vi "serial_communication.vi"() -> ()   [LabVIEW 2017]
uses:
  Utility Sub VIs/diode_charts.ctl
  <vilib>/Instr/_visa.llb/VISA Set IO Buffer Mask.ctl
  <vilib>/Instr/_visa.llb/VISA Flush IO Buffer Mask.ctl
  <vilib>/Instr/_visa.llb/VISA Configure Serial Port (Instr).vi
panel:
  out "read buffer":string
  in  "stop":bool
  in  "VISA resource name":refnum<visa-resource-name>
  out "value":T1
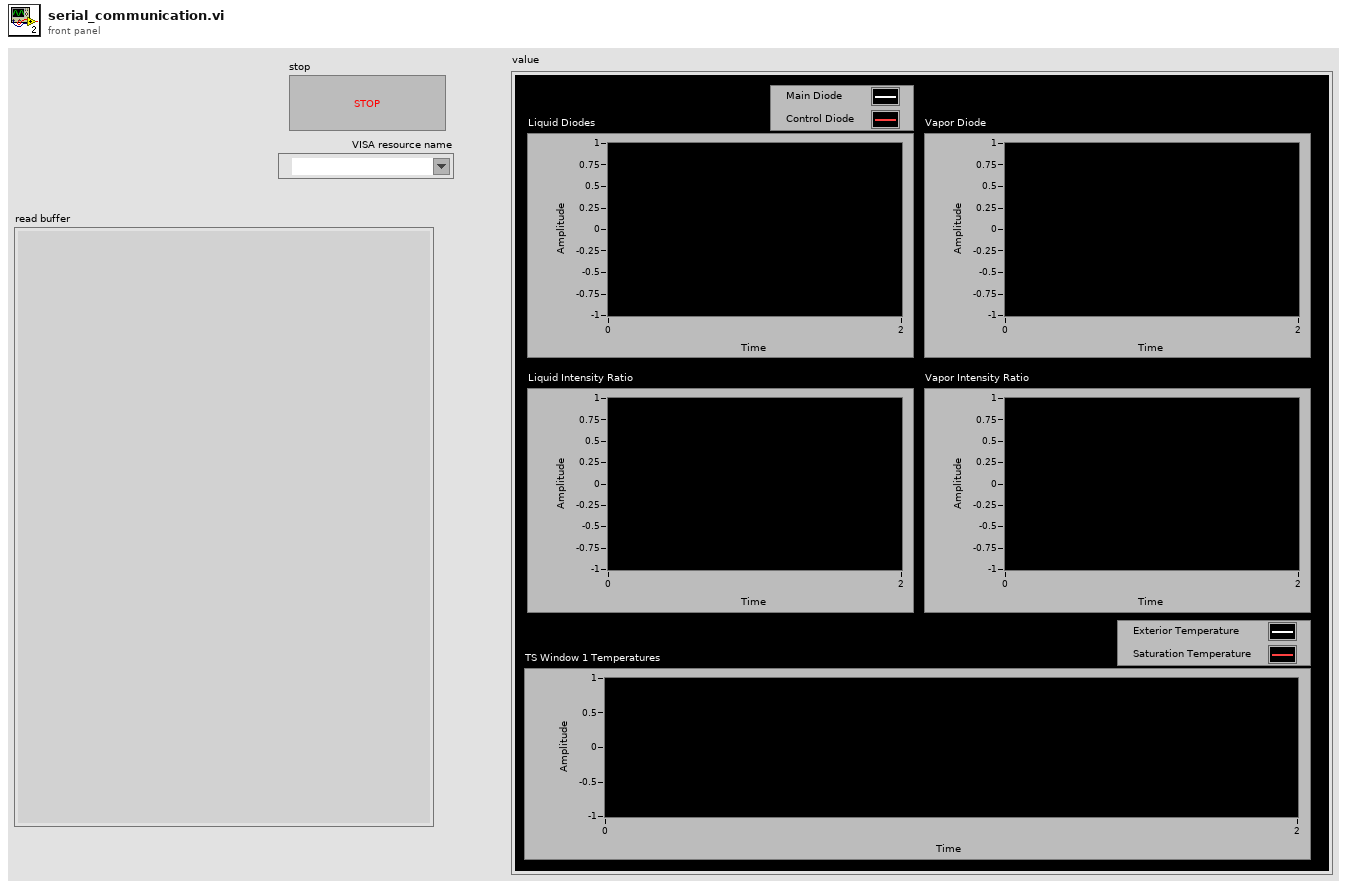
[diagram p1: front panel]
types:
  T1 = typedef "diode_charts.ctl" = cluster{"Liquid Diodes":cluster{dbl, dbl}, "Liquid Intensity Ratio":dbl, "Vapor Diode":cluster{dbl, dbl}, "Vapor Intensity Ratio":dbl, "TS Window 1 Temperatures":cluster{"Average":dbl, "T Sat [C]":dbl}}
  T2 = typedef "VISA Set IO Buffer Mask.ctl" = u16
  T3 = typedef "VISA Flush IO Buffer Mask.ctl" = u16
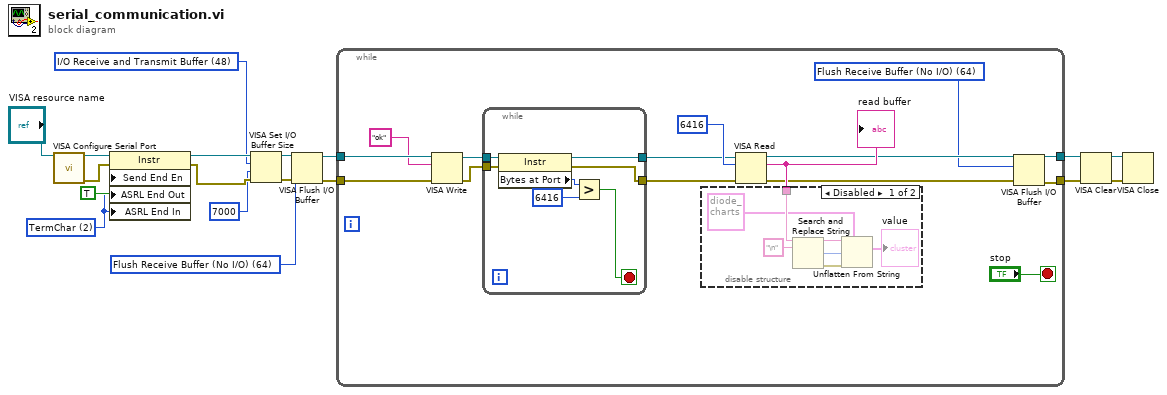
[diagram p0: block diagram]
diagram:
  w2 = T2 48 items=["I/O Receive Buffer"=16, "I/O Transmit Buffer"=32, "I/O Receive and Transmit Buffer"=48] ("Mask")
  w8 = T3 64 items=["Flush Receive Buffer"=16, "Write Transmit Buffer to Device"=32, "Flush Receive Buffer (No I/O)"=64, "Flush Transmit Buffer"=128] ("Mask")
  w11 = u16 2 items=["None", "Last Bit", "TermChar", "Break"] ("Serial Settings:End Mode for Writes")
  n1 = call-poly "VISA Configure Serial Port"("VISA resource name"="VISA resource name") -> ("VISA resource name out"=w14:refnum<visa-resource-name>, "error out"=w13:errorcluster)  [unwired: 13 in]
  n2 = property class="Instr"(reference=w14, error in=w13, "Send End En"=TRUE ("Message Based Settings:Send End Enable"), "ASRL End Out"=w11, "ASRL End In"=w11) -> (reference out=w4:refnum<visa-resource-name>, error out=w3:errorcluster)
  n3 = VISA Set I/O Buffer Size(VISA resource name=w4, mask (16)=w2, size (4096)=u32 7000, error in (no error)=w3) -> (VISA resource name out=w5:refnum<visa-resource-name>, error out=w6:errorcluster)
  n4 = VISA Flush I/O Buffer(VISA resource name=w5, mask (16)=w8, error in (no error)=w6) -> (VISA resource name out=w9:refnum<visa-resource-name>, error out=w7:errorcluster)
  n5 = while {
    tunnel: w9 -> [w32]
    tunnel: w7 -> [w31]
    tunnel: [w22] -> w17
    tunnel: [w23] -> w18
    stop <- "stop" stop-if-true
    w19 = T3 64 items=["Flush Receive Buffer"=16, "Write Transmit Buffer to Device"=32, "Flush Receive Buffer (No I/O)"=64, "Flush Transmit Buffer"=128] ("Mask")
    n6 = VISA Write(VISA resource name=w32, write buffer="ok", error in (no error)=w31) -> (VISA resource name out=w27:refnum<visa-resource-name>, error out=w26:errorcluster)  [unwired: 1 out]
    n7 = while {
      tunnel: w27 -> [w40]
      tunnel: w26 -> [w39]
      tunnel: [w35] -> w25
      tunnel: [w34] -> w24
      stop <- w36 stop-if-true
      n8 = property class="Instr"(reference=w40, error in=w39) -> (reference out=w35:refnum<visa-resource-name>, error out=w34:errorcluster, "Bytes at Port"=w38:u32)
      n9 = Greater?(x=w38, y=u32 6416) -> (0:w36:bool)
    }
    n10 = VISA Read(VISA resource name=w25, byte count=u32 6416 ("y"), error in (no error)=w24) -> (VISA resource name out=w21:refnum<visa-resource-name>, read buffer=w29:string, error out=w20:errorcluster)  [unwired: 1 out]
    "read buffer" <- w29
    n11 = disable-structure shown="Disabled" {
      disable-tunnel: w29 -> [w47 _]
      frame Disabled {
        n12 = Search and Replace String(input string=w47, search string="\n") -> (result string=w43:string, number of replacements=w44:i32, error out=w45:errorcluster)  [unwired: 6 in, 1 out]
        n13 = Unflatten From String(type=T1 {"Liquid Diodes"={0.0, 0.0}, "Liquid Intensity Ratio"=0.0, "Vapor Diode"={0.0, 0.0}, "Vapor Intensity Ratio"=0.0, "TS Window 1 Temperatures"={"Average"=0.0, "T Sat [C]"=0.0}} ("notification"), binary string=w43, byte order (0:big-endian, network order)=w44, error in (no error)=w45) -> (value=→"value":T1)  [unwired: 1 in, 2 out]
      }
      frame Enabled {
      }
    }
    n14 = VISA Flush I/O Buffer(VISA resource name=w21, mask (16)=w19, error in (no error)=w20) -> (VISA resource name out=w22:refnum<visa-resource-name>, error out=w23:errorcluster)
  }
  n15 = VISA Clear(VISA resource name=w17, error in (no error)=w18) -> (VISA resource name out=w15:refnum<visa-resource-name>, error out=w16:errorcluster)
  n16 = VISA Close(VISA resource name=w15, error in (no error)=w16) -> ()  [unwired: 1 out]
